vi "Inter Face.vi"() -> ()   [LabVIEW 2015]
uses:
  GUI_Control/Alarm.ctl
  GUI_Control/Home.ctl
  GUI_Control/Login.ctl
  GUI_Control/Manual.ctl
  GUI_Control/Open_data.ctl
  GUI_Control/Pause.ctl
  GUI_Control/Start.ctl
  GUI_Control/Stop.ctl
  GUI_Control/Inforamation_11.ctl
  <userlib>/QMH/Message Queue/Support/RunType.ctl
  <userlib>/QMH/Message Queue/Support/Enqueue Message (Single).vi
  <vilib>/Utility/error.llb/Error Cluster From Error Code.vi
  <userlib>/QMH/Message Queue/Support/Enqueue Message (Array).vi
  <userlib>/QMH/Message Queue/Support/Run Module(ref).vi
  <vilib>/ErrorRing/Error Ring.xnode
  <userlib>/QMH/User Event - Stop/User Event - Stop.lvlib
  <userlib>/QMH/Message Queue/Message Queue.lvlib
panel:
  out "输出数组":string[](array[string])
  out "权限":enum16{"学生", "老师"}(ring)
  out "Time":string
  out "Data":string
  in  "Machine Information":T1
  in  "Exit":T2
  in  "Start":T3 caption="进入Scada监控"
  in  "Pause":T4
  in  "OpenData":T5 caption="动作-告警监视"
  in  "Manual":T6 caption="遥信遥测监控"
  in  "User":T7 caption="用户操作"
  in  "HOME":T8 caption="进入待机界面"
  in  "Alarm Information":T9
  in  "HostThread":variant
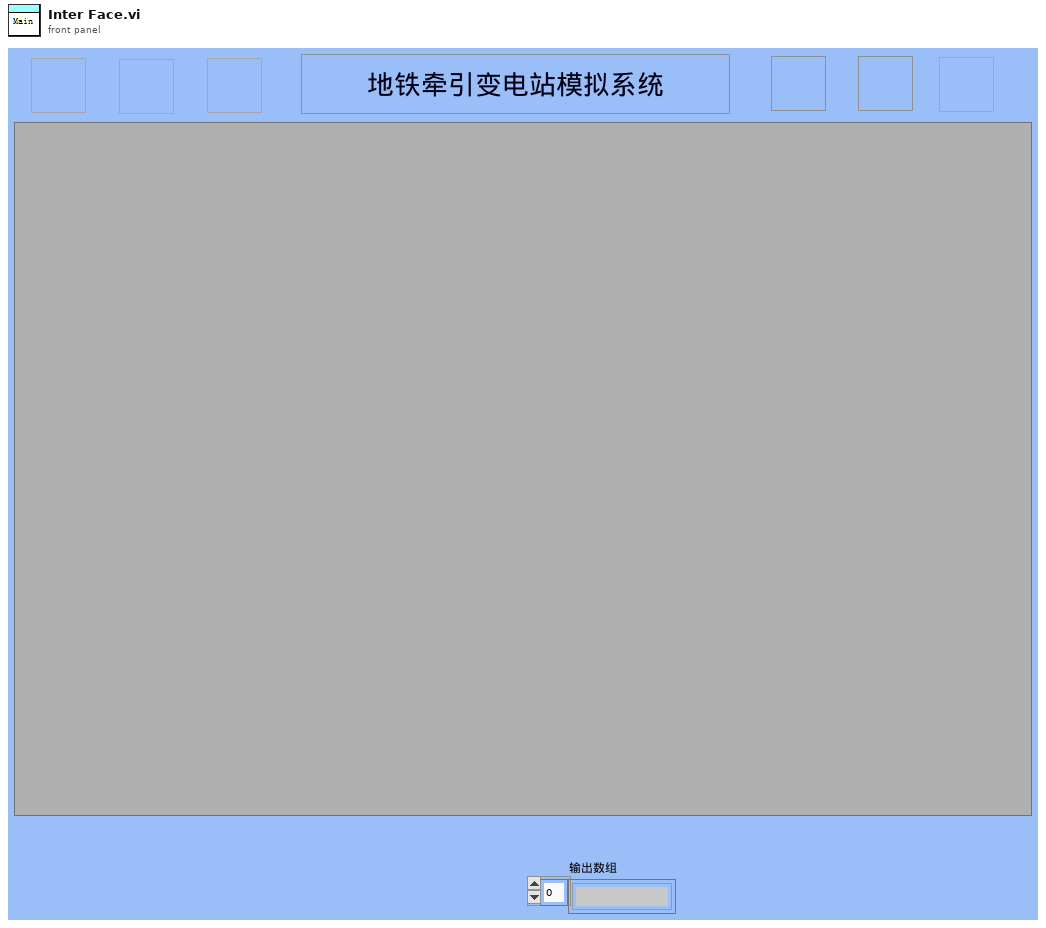
[diagram p1: front panel]
types:
  T1 = typedef "Inforamation_11.ctl" = bool
  T2 = typedef "Stop.ctl" = bool
  T3 = typedef "Start.ctl" = bool
  T4 = typedef "Pause.ctl" = bool
  T5 = typedef "Open_data.ctl" = bool
  T6 = typedef "Manual.ctl" = bool
  T7 = typedef "Login.ctl" = bool
  T8 = typedef "Home.ctl" = bool
  T9 = typedef "Alarm.ctl" = bool
  T10 = cluster{"Controls":cluster{"Exit":refnum<vi>, "Start":refnum<vi>, "Pause":refnum<vi>, "OpenData":refnum<vi>, "Machine Information":refnum<vi>, "Manual":refnum<vi>, "User":refnum<vi>, "HOME":refnum<vi>, "Alarm Information":refnum<vi>}, "Thread":cluster{"ThisQ":string, "ThisVI":refnum<vi>, "HostQ":string, "HostRef":refnum<vi>, "SlavesQ":string[], "SlavesRef":refnum<vi>[]}, "Data":cluster{"Replace":bool}, "User":cluster{"Name":string}, "子面板":refnum<vi>, " Authority":enum16{"学生", "老师"}}
  T11 = enum32{"Invalid", "Standard", "Closed", "Hidden", "Minimized", "Maximized"}
  T12 = typedef "Message Queue.lvlib/RunType.ctl" = enum16{"Embeded", "Standard", "Hidden", "Minimized", "Maximzed", "RealTime"}
  T13 = enum8{"Enabled", "Disabled", "Disabled and Grayed Out"}
  T14 = cluster{"Exit":refnum<vi>, "Start":refnum<vi>, "Pause":refnum<vi>, "OpenData":refnum<vi>, "Machine Information":refnum<vi>, "Manual":refnum<vi>, "User":refnum<vi>, "HOME":refnum<vi>, "Alarm Information":refnum<vi>}
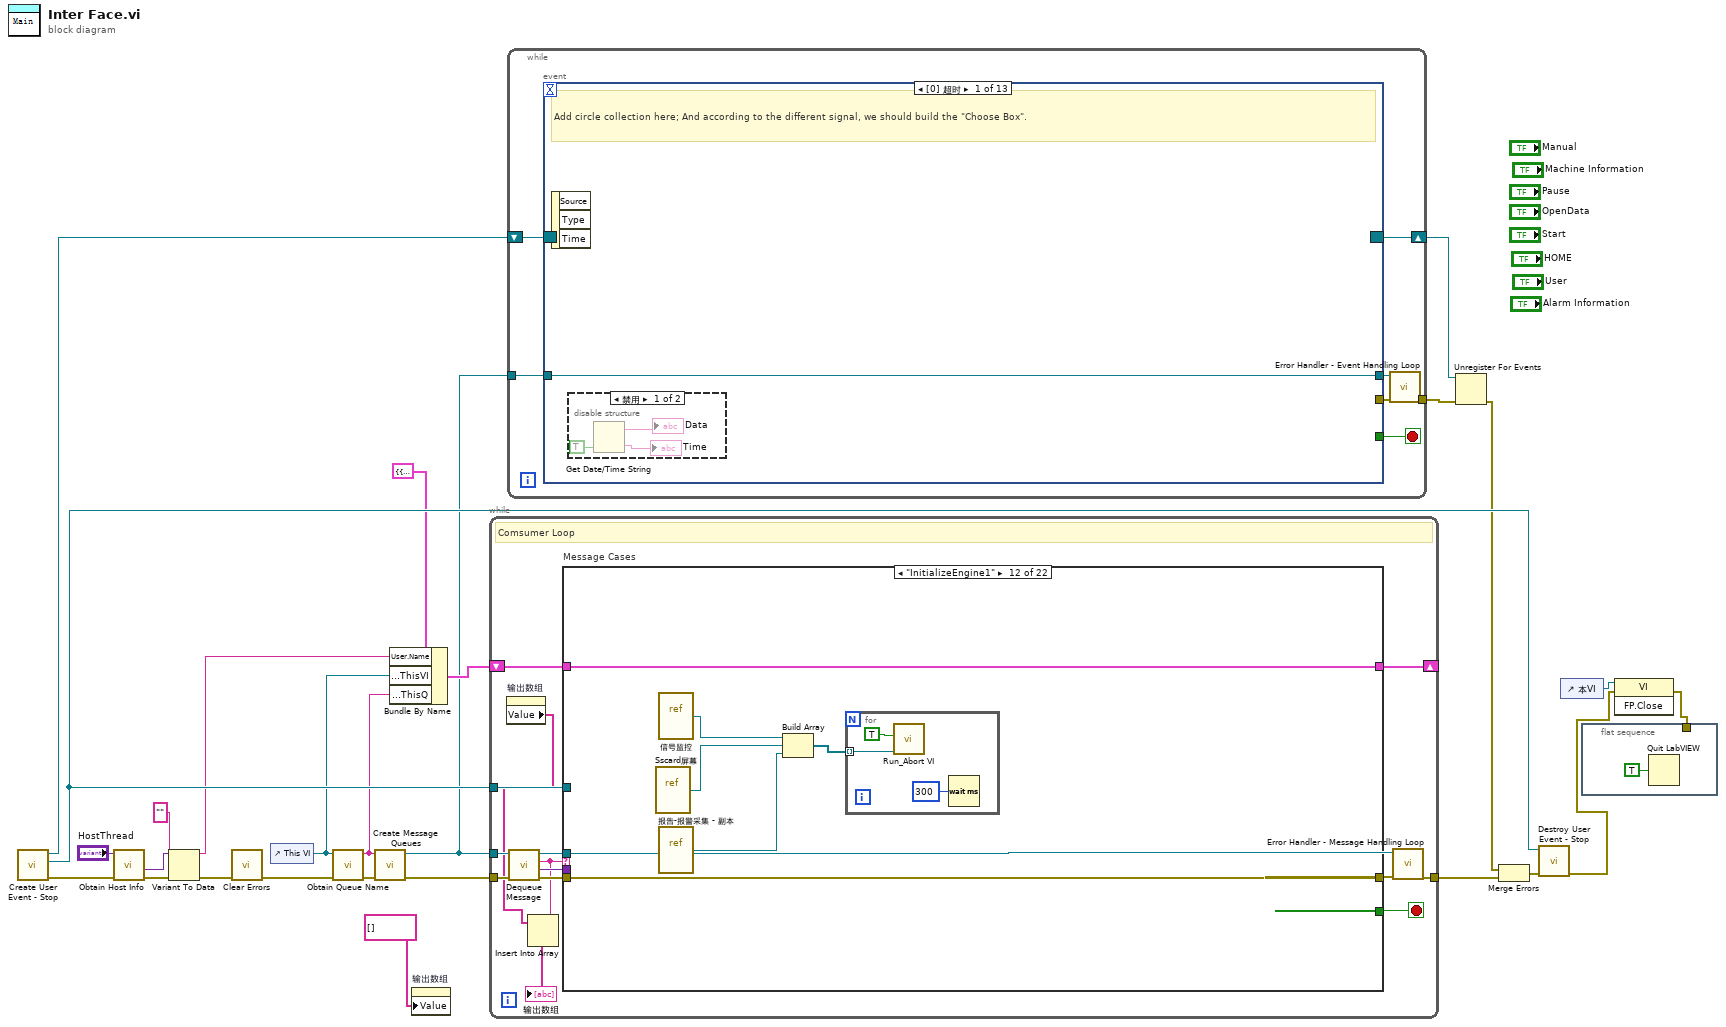
[diagram p0: block diagram]
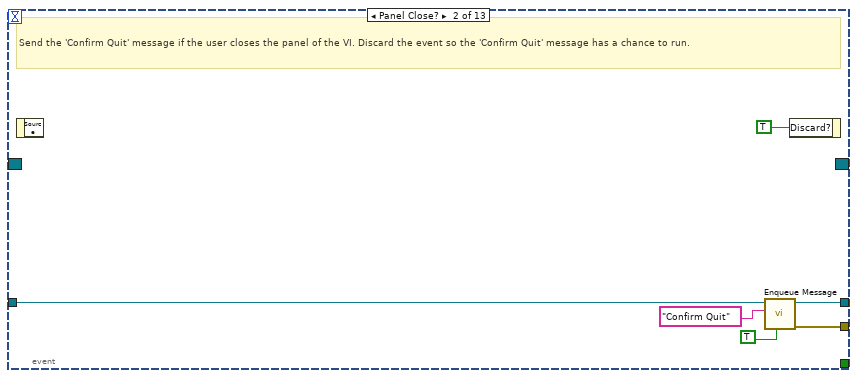
[diagram p3: hidden frame]
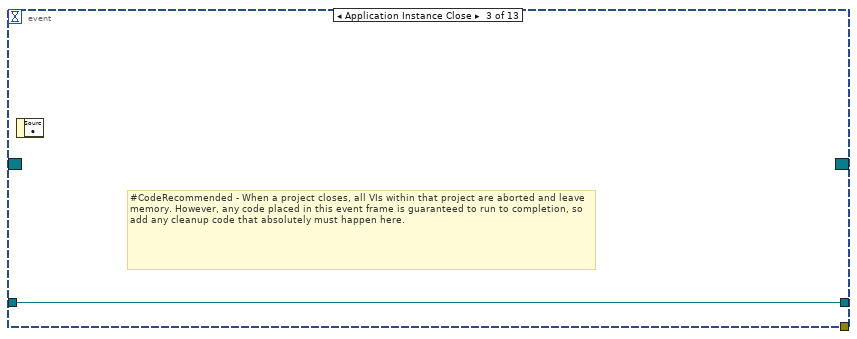
[diagram p4: hidden frame]
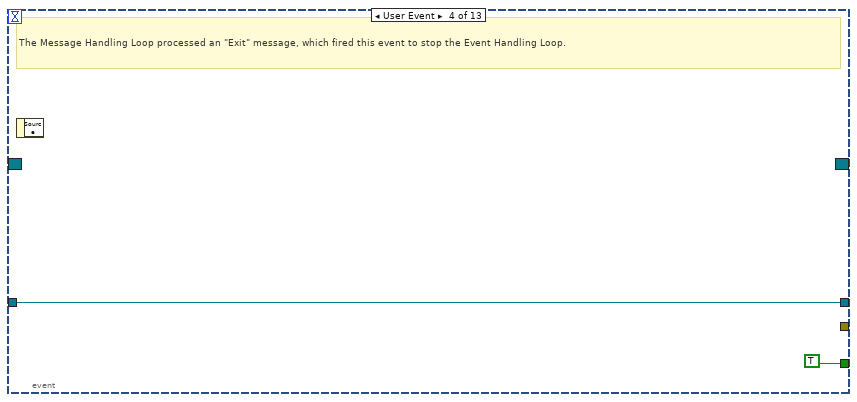
[diagram p5: hidden frame]
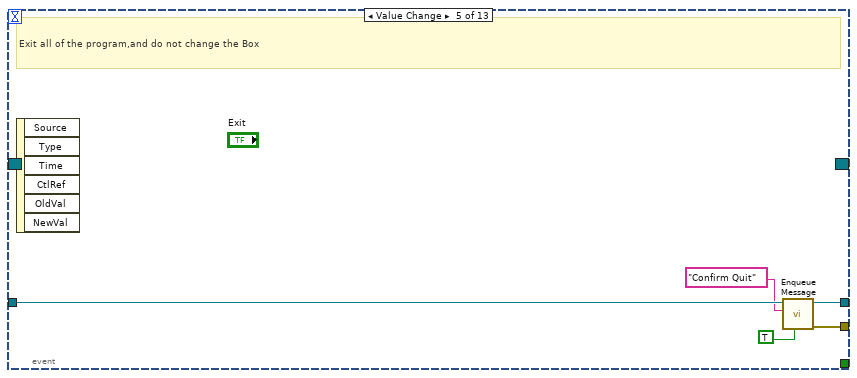
[diagram p6: hidden frame]
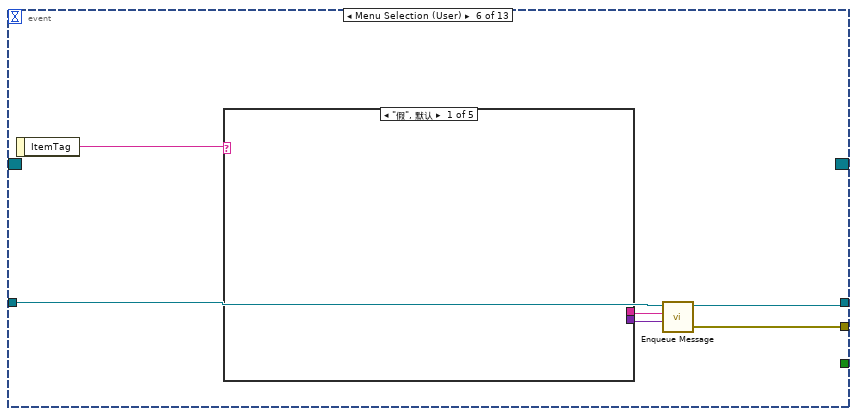
[diagram p7: hidden frame]
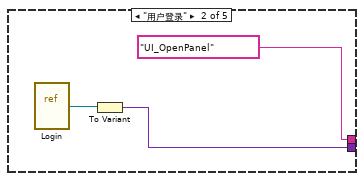
[diagram p8: hidden frame]
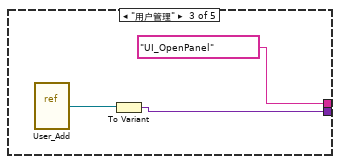
[diagram p9: hidden frame]
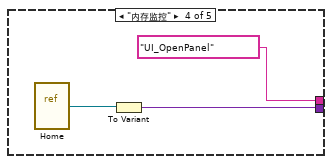
[diagram p10: hidden frame]
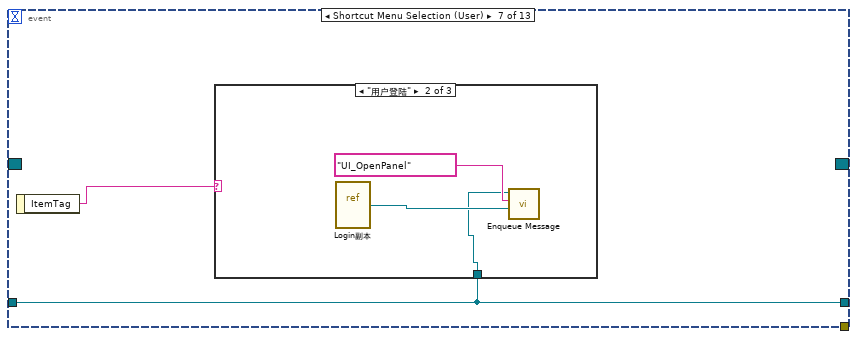
[diagram p12: hidden frame]
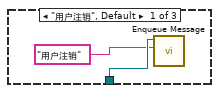
[diagram p13: hidden frame]
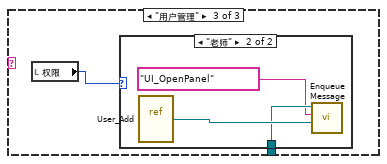
[diagram p14: hidden frame]
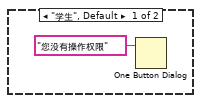
[diagram p15: hidden frame]
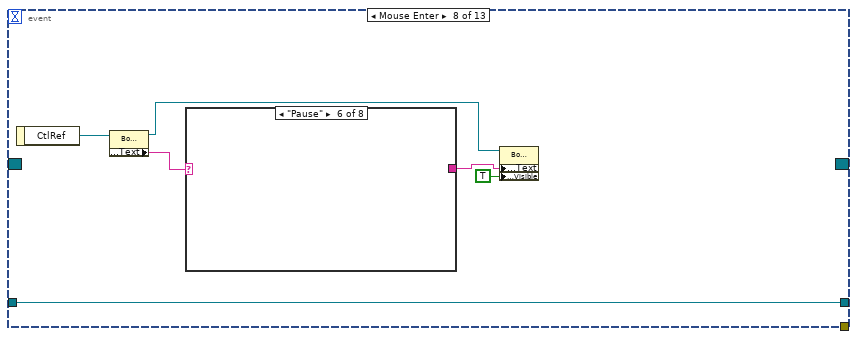
[diagram p16: hidden frame]
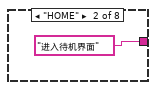
[diagram p18: hidden frame]
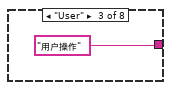
[diagram p19: hidden frame]
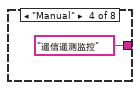
[diagram p20: hidden frame]
diagram:
  n1 = call <userlib>:"Create User Event - Stop.vi"() -> ("error out"=w14:errorcluster, "User Event - Stop"=w22:refnum<user-event>, "Stop Event Registration Refnum"=w24:refnum<event-registration>)  [unwired: 9 in]
  n2 = call <userlib>:"Obtain Host Info.vi"("error in (no error)"=w14, "HostThread"="HostThread") -> ("error out"=w11:errorcluster, "Data"=w10:variant)  [unwired: 6 in, 2 out]
  n3 = Variant To Data(error in=w11, type="", Variant=w10) -> (data=w6:string, error out=w8:errorcluster)
  n4 = call <vilib>:"Clear Errors.vi"("error in (no error)"=w8) -> ("error out"=w7:errorcluster)  [unwired: 5 in, 1 out]
  n5 = control-ref of="This VI"() -> (w5:refnum<vi>)
  n6 = call <userlib>:"Obtain Queue Name.vi"("error in (no error)"=w7, "VI Refnum"=w5) -> ("error out"=w18:errorcluster, "ViName"=w15:string)  [unwired: 8 in]
  n7 = call <userlib>:"Create Message Queues.vi"("error in (no error)"=w18, "name (unnamed)"=w15) -> ("error out"=w26:errorcluster, "QueueHandler"=w12:refnum<queue>)  [unwired: 8 in]
  n8 = Bundle By Name(cluster=T10 {"Controls"={"Exit"=refnum, "Start"=refnum, "Pause"=refnum, "OpenData"=refnum, "Machine Information"=refnum, "Manual"=refnum, "User"=refnum, "HOME"=refnum, "Alarm Information"=refnum}, "Thread"={"ThisQ"="", "ThisVI"=refnum, "HostQ"="", "HostRef"=refnum, "SlavesQ"=[], "SlavesRef"=[]}, "Data"={"Replace"=FALSE}, "User"={"Name"=""}, "子面板"=refnum, " Authority"=enum."学生"} ("Data Cluster"), "User.Name"=w6, "Thread.ThisVI"=w5, "Thread.ThisQ"=w15) -> (w16:T10)
  n9 = property on="输出数组" class="Arr (严格)"("Value"=string[] []) -> ()  [unwired: 2 in, 2 out]
  n10 = while {
    tunnel: w12 -> [w33]
    shift-right: [w39] -> _
    shift-left: w16 -> [w40]
    tunnel: w22 -> [w37]
    tunnel: w26 -> [w36]
    tunnel: [w31] -> w25
    stop <- w38 stop-if-true
    # "Comsumer Loop"
    n11 = property on="输出数组" class="Arr (严格)"() -> ("Value"=w27:string[])  [unwired: 2 in, 2 out]
    n12 = call <userlib>:"Dequeue Message.vi"("error in (no error)"=w36, "Message Queue"=w33) -> ("error out"=w35:errorcluster, "Message Data"=w34:variant, "Message"=w29:string, "dup Message Queue"=w32:refnum<queue>)  [unwired: 6 in]
    n13 = Insert Into Array(array=w27, new element=w29) -> (→"输出数组":string[])  [unwired: 1 in]
    n14 = case "Message Cases" shown="\"InitializeEngine1\"" w29 {
      selector: w29 -> [w41 _ _ _ _ _ _ _ _ _ _ _ _ _ _ _ _ _ _ _ _ _]
      tunnel: w32 -> [_ w59 _ w75 w89 _ w100 _ _ _ _ _ _ _ _ _ _ _ _ _ _ _]
      tunnel: w35 -> [_ w56 w73 w81 w87 w91 w102 w105 w111 w125 w137 w146 w151 w165 w177 w182 w193 w199 w201 w202 w205 w216]
      tunnel: [w42 w51 w68 w79 w88 w91 w101 w105 w111 w125 w137 w146 w151 w165 w177 w182 w193 w199 w201 w202 w205 w216] -> w30
      tunnel: w40 -> [w43 w53 w65 w80 w90 w92 w98 w104 w107 w124 w136 w145 w150 w164 w166 w181 w190 w196 w200 w203 w204 w215]
      tunnel: [w43 w53 w65 w80 w90 w92 w97 w104 w107 w124 w136 w145 w150 w163 w166 w181 w190 w196 w200 w203 w204 w215] -> w39
      tunnel: [_ TRUE _ _ _ _ _ _ _ _ _ _ _ _ _ _ _ _ _ _ _ _] -> w38
      tunnel: w34 -> [_ _ w72 _ _ _ w99 _ _ _ _ _ _ _ _ _ w192 w198 _ _ _ _]
      tunnel: w37 -> [_ w55 _ _ _ _ _ _ _ _ _ _ _ _ _ _ _ _ _ _ _ _]
      frame Default {
        # "'Default' case only runs if there is a message that isn't defined in any of the other cases.  Output a programming error."
        n15 = xnode "Error Ring"("参数 0"=w41) -> ("错误输出"=w42:errorcluster)
      }
      frame "Exit" {
        # "Stop the VI"
        # "Release the message queue reference"
        # "#CodeNeeded - Add any required cleanup code here"
        # "Exit - Exit the application."
        n16 = call <userlib>:"Fire User Event - Stop.vi"("User Event - Stop"=w55) -> ("error out"=w54:errorcluster)  [unwired: 10 in]
        n17 = Release Queue(queue=w59, error in (no error)=w56) -> (error out=w57:errorcluster)  [unwired: 1 in, 2 out]
        n18 = Merge Errors(w54, w57) -> (w51:errorcluster)
        n19 = call "Loop.vi"("Loop"=enum16{"Do Nothing", "Loop", "Stop"}."Stop") -> ()  [unwired: 4 in, 1 out]
      }
      frame "Error" {
        # "Error - Check the error message data and respond accordingly. This message is sent by the \"Error Handler\" VIs at the end of each loop in this application."
        n20 = Unbundle By Name(w65) -> ("Thread.HostQ"=w64:string)
        n21 = Variant To Data(error in=w73, type=errorcluster {"status"=FALSE, "code"=0, "source"=""} ("error constant"), Variant=w72) -> (data=w61:errorcluster, error out=w70:errorcluster)
        n22 = To Variant(anything=w61) -> (Variant=w60:variant)
        n23 = call <userlib>:"Obtain Message Queue.vi"("name (unnamed)"=w64) -> ("error out"=w63:errorcluster, "Message Queue"=w62:refnum<queue>)  [unwired: 9 in]
        n24 = call-poly <userlib>:"Enqueue Message.vi"("Priority Message? (F)"=TRUE, "error in (no error)"=w63, "Message Data"=w60, "Message"="Error", "Message Queue"=w62) -> ("error out"=w69:errorcluster)  [unwired: 5 in, 1 out]
        n25 = Merge Errors(w69, w70) -> (w68:errorcluster)
      }
      frame "Confirm Quit" {
        # "Confirm Quit - Message that can confirm whether or not the user wants to exit the application."
        n26 = for {
          tunnel: string[] ["Home.vi", "Sscard屏幕.vi", "AlarmInterFace.vi", "继保.vi", "测试接收队列.vi", "灯组解析.vi"] -> [w83] mode=indexing
          n27 = call <userlib>:"Obtain Message Queue.vi"("name (unnamed)"=w83) -> ("Message Queue"=w84:refnum<queue>)  [unwired: 9 in, 1 out]
          n28 = call-poly <userlib>:"Enqueue Message.vi"("Priority Message? (F)"=TRUE, "Message"="Exit", "Message Queue"=w84) -> ()  [unwired: 7 in, 2 out]
        }
        n29 = call-poly <userlib>:"Enqueue Message.vi"("Priority Message? (F)"=TRUE, "error in (no error)"=w81, "Message"="Exit", "Message Queue"=w75) -> ("error out"=w78:errorcluster)  [unwired: 6 in, 1 out]
        n30 = Merge Errors(w78) -> (w79:errorcluster)
      }
      frame "Initialize" {
        # "Initialize - Send separate messages to initialize the data and the front panel.  Bundle control references."
        n31 = call-poly <userlib>:"Enqueue Message.vi"("error in (no error)"=w87, "Message Array"=string[] ["UI_InitContorlRef", "UI_InitializePanel", "User_Initialize", "UI_InitContorlVal"], "Message Queue"=w89) -> ("error out"=w88:errorcluster)  [unwired: 7 in, 1 out]
      }
      frame "<-------User-------->" {
      }
      frame "User_Initialize" {
        w94 = enum16{"学生", "老师"}."学生"  # Authority
        n32 = Variant To Data(type=w94, Variant=w99) -> (data=w93:enum16{"学生", "老师"}, error out=w96:errorcluster)  [unwired: 1 in]
        "权限" <- w93
        n33 = call <vilib>:"Clear Errors.vi"("error in (no error)"=w96) -> ()  [unwired: 5 in, 2 out]
        n34 = Bundle By Name(cluster=w98, "Authority"=w93) -> (w97:T10)
        n35 = call "Loop.vi"("Loop"=enum16{"Do Nothing", "Loop", "Stop"}."Loop") -> ()  [unwired: 4 in, 1 out]
        n36 = call-poly <userlib>:"Enqueue Message.vi"("error in (no error)"=w102, "Message Array"=string[] ["User_Wirte authority", "User_update authority1", "User_update authority2", "InitializeEngine", "InitializeEngine1"], "Message Queue"=w100) -> ("error out"=w101:errorcluster)  [unwired: 7 in, 1 out]
      }
      frame "User_Wirte authority" {
      }
      frame "User_update authority1" {
        n37 = Unbundle By Name(w107) -> ("Authority"=w106:enum16{"学生", "老师"})
        n38 = case shown="\"学生\", 默认" w106 {
          tunnel: [bool[] [FALSE] _] -> w109
          frame "学生", Default {
          }
          frame "老师" {
          }
        }
        n39 = Current VI's Menubar() -> (w110:refnum<k9>)
        n40 = for {
          tunnel: w110 -> [w114]
          tunnel: w109 -> [w113] mode=indexing
          tunnel: string[] ["用户管理"] -> [w112] mode=indexing
          n41 = Set Menu Item Info(7:w112, 9:w113, 10:w112, 11:w114) -> ()  [unwired: 3 in, 2 out]
        }
      }
      frame "User_update authority2" {
        n42 = Unbundle By Name(w124) -> ("Controls.Exit"=w118:refnum<vi>, "Controls.OpenData"=w123:refnum<vi>, "Controls.HOME"=w122:refnum<vi>, "Controls.Manual"=w121:refnum<vi>, "Controls.Start"=w117:refnum<vi>, "Authority"=w116:enum16{"学生", "老师"})
        n43 = Build Array(w118, w123, w122, w121, w117) -> (w120:refnum<vi>[])
        n44 = case shown="\"学生\", 默认" w116 {
          tunnel: [i32[] [2, 2, 2, 2, 0] i32[] [0, 0, 0, 0, 0]] -> w119
          frame "学生", Default {
          }
          frame "老师" {
          }
        }
        n45 = for {
          tunnel: w120 -> [w127] mode=indexing
          tunnel: w119 -> [w126] mode=indexing
          n46 = property class="Bool"(reference=w127, "DisabledEnum"=w126) -> ()  [unwired: 1 in, 2 out]
        }
      }
      frame "InitializeEngine" {
        n47 = vi-ref "管理机.vi"() -> (w135:refnum<vi>)
        n48 = vi-ref "继保.vi"() -> (w133:refnum<vi>)
        n49 = vi-ref "OPC.vi"() -> (w132:refnum<vi>)
        n50 = vi-ref "测试接收队列.vi"() -> (w131:refnum<vi>)
        n51 = vi-ref "灯组解析.vi"() -> (w130:refnum<vi>)
        n52 = Build Array(w135, w133, w132, w131, w130) -> (w134:refnum<vi>[])
        n53 = for {
          tunnel: w134 -> [w139] mode=indexing
          n54 = call "Run_Abort VI.vi"("VI引用句柄"=w139, "Run?(Default Abort)"=TRUE) -> ()  [unwired: 10 in]
          n55 = Wait (ms)(milliseconds to wait=u32 300 ("等待时间（毫秒）")) -> ()  [unwired: 1 out]
        }
      }
      frame "InitializeEngine1" {
        n56 = vi-ref "Sscard屏幕.vi"() -> (w142:refnum<vi>)
        n57 = vi-ref "信号监控.vi"() -> (w143:refnum<vi>)
        n58 = vi-ref "报告-报警采集 - 副本.vi"() -> (w141:refnum<vi>)
        n59 = Build Array(w143, w142, w141) -> (w144:refnum<vi>[])
        n60 = for {
          tunnel: w144 -> [w148] mode=indexing
          n61 = call "Run_Abort VI.vi"("VI引用句柄"=w148, "Run?(Default Abort)"=TRUE) -> ()  [unwired: 10 in]
          n62 = Wait (ms)(milliseconds to wait=u32 300 ("等待时间（毫秒）")) -> ()  [unwired: 1 out]
        }
      }
      frame "<-------UI-------->" {
      }
      frame "UI_InitContorlRef" {
        n63 = control-ref of="Exit"() -> (w162:refnum<vi>)
        n64 = control-ref of="Start"() -> (w161:refnum<vi>)
        n65 = control-ref of="Pause"() -> (w160:refnum<vi>)
        n66 = control-ref of="HOME"() -> (w155:refnum<vi>)
        n67 = control-ref of="Alarm Information"() -> (w154:refnum<vi>)
        n68 = control-ref of="OpenData"() -> (w159:refnum<vi>)
        n69 = control-ref of="Manual"() -> (w157:refnum<vi>)
        n70 = control-ref of="User"() -> (w156:refnum<vi>)
        n71 = control-ref of="Machine Information"() -> (w158:refnum<vi>)
        n72 = Bundle("Exit"=w162, "Start"=w161, "Pause"=w160, "OpenData"=w159, "Machine Information"=w158, "Manual"=w157, "User"=w156, "HOME"=w155, "Alarm Information"=w154) -> (w153:T14)  [unwired: 1 in]
        n73 = control-ref of="子面板"() -> (w152:refnum<vi>)
        n74 = Bundle By Name(cluster=w164, "Controls"=w153, "子面板"=w152) -> (w163:T10)
      }
      frame "UI_InitContorlVal" {
        # "初始化控件值"
        n75 = Unbundle By Name(w166) -> ("Controls.Machine Information"=w175:refnum<vi>, "Controls.Exit"=w174:refnum<vi>, "Controls.Start"=w173:refnum<vi>, "Controls.Pause"=w172:refnum<vi>, "Controls.OpenData"=w171:refnum<vi>, "Controls.Manual"=w170:refnum<vi>, "Controls.User"=w169:refnum<vi>, "Controls.HOME"=w168:refnum<vi>)
        n76 = Build Array(w174, w173, w172, w171, w170, w169, w168) -> (w167:refnum<vi>[])
        n77 = for {
          tunnel: w167 -> [w178] mode=indexing
          n78 = invoke class="Bool" method="Reinit To Default"(reference=w178) -> ()  [unwired: 2 in, 3 out]
        }
        n79 = property class="Bool (严格)"(reference=w175, "BoolText.Text"="地铁牵引变电站模拟系统" ("布尔文本.文本")) -> ()  [unwired: 1 in, 2 out]
      }
      frame "UI_InitializePanel" {
        # "加载初始子面板VI"
        n80 = Unbundle By Name(w181) -> ("子面板"=w180:refnum<vi>)
        n81 = vi-ref "Home.vi"() -> (w179:refnum<vi>)
        n82 = call "Serch.vi"("静态VI"=w179, "子面板"=w180) -> ()  [unwired: 2 in]
      }
      frame "UI_OpenPanel" {
        # "运行VI，如果状态为运行，打开前面板， 在子VI中设置退出时候是否结束程序"
        n83 = Variant To Data(type=refnum<vi> refnum, Variant=w192) -> (data=w189:refnum<vi>)  [unwired: 1 in, 1 out]
        n84 = call-poly <userlib>:"Run Module.vi"("Type"=RunType."Standard", "VI Ref in"=w189) -> ("VI Ref out"=w183:refnum<vi>)  [unwired: 7 in, 2 out]
        n85 = invoke class="VI" method="FP.Open"(reference=w183, "Activate"=TRUE ("激活？"), "State"=T11."Standard" ("状态")) -> (reference out=w187:refnum<vi>)  [unwired: 2 in, 4 out]
        n86 = property class="VI"(reference=w187, "Front Panel.IsFrontmost"=TRUE ("前面板窗口:在最前")) -> ()  [unwired: 1 in, 2 out]
      }
      frame "UI_insertPanel" {
        # "VI插入子面板"
        n87 = Unbundle By Name(w196) -> ("子面板"=w195:refnum<vi>)
        n88 = Variant To Data(type=refnum<vi> refnum, Variant=w198) -> (data=w194:refnum<vi>)  [unwired: 1 in, 1 out]
        n89 = call "Serch.vi"("静态VI"=w194, "子面板"=w195) -> ()  [unwired: 2 in]
      }
      frame "<------Core------>" {
      }
      frame "Core_InitializeRef" {
        # "Initialize control references. For there is not enough space to locate all the control references, separate the codes into 2 messages"
      }
      frame "<---Operation--->" {
      }
      frame "用户注销" {
        n90 = Unbundle By Name(w215) -> ("Controls.OpenData"=w212:refnum<vi>, "Controls.Manual"=w211:refnum<vi>, "Controls.Alarm Information"=w210:refnum<vi>, "Controls.Start"=w209:refnum<vi>, "子面板"=w207:refnum<vi>)
        n91 = vi-ref "Home.vi"() -> (w208:refnum<vi>)
        n92 = Build Array(w212, w211, w210, w209) -> (w214:refnum<vi>[])
        n93 = call "Serch.vi"("静态VI"=w208, "子面板"=w207) -> ()  [unwired: 2 in]
        n94 = for {
          tunnel: w214 -> [w218] mode=indexing
          tunnel: T13."Disabled and Grayed Out" ("禁用") -> [w217]
          n95 = property class="Bool (严格)"(reference=w218, "DisabledEnum"=w217) -> ()  [unwired: 1 in, 2 out]
        }
        n96 = local write "权限"(enum16{"学生", "老师"}."学生" ("权限")) -> ()
      }
    }
    n97 = call <userlib>:"Error Handler - Message Handling Loop.vi"("error in (no error)"=w30, "Message Queue"=w32) -> ("dup error in"=w31:errorcluster)  [unwired: 8 in, 1 out]
  }
  n98 = while {
    tunnel: w12 -> [w225]
    shift-right: [w223] -> w20
    shift-left: w24 -> [w224]
    tunnel: [w219] -> w19
    stop <- w221 stop-if-true
    # "Producer Loop"
    n99 = event shown="[0] 超时" {
      selector: w224 -> [_ _ _ _ _ _ _ _ _ _ _ _ _]
      dyn-events: [_ _ _ _ _ _ _ _ _ _ _ _ _] -> w223
      timeout: _ -> [_ _ _ _ _ _ _ _ _ _ _ _ _]
      tunnel: [_ _ _ TRUE ("Discard?") _ _ _ _ _ _ _ _ _] -> w221
      tunnel: w225 -> [w226 w234 w236 w238 w243 w247 w259 w277 w285 w289 w298 w307 w316]
      tunnel: [_ w233 _ _ w241 w248 _ _ _ _ _ _ _] -> w222
      tunnel: [w226 w232 w236 w238 w242 w249 w259 w277 w285 w288 w297 w305 w315] -> w220
      event Timeout {
        # "Add circle collection here; And according to the different signal, we should build the \"Choose Box\"."
        n100 = event-data() -> ()  [unwired: 1 in, 3 out]
        n101 = disable-structure shown="禁用" {
          frame Disabled {
            n102 = Get Date/Time String(want seconds? (F)=TRUE ("需要秒？(F)")) -> (date string=→"Data":string, time string=→"Time":string)  [unwired: 2 in]
          }
          frame Enabled {
          }
        }
      }
      event Panel Close? {
        # "Send the 'Confirm Quit' message if the user closes the panel of the VI. Discard the event so the 'Confirm Quit' message has a chance to run."
        n103 = event-data() -> ()  [unwired: 1 in, 1 out]
        n104 = call-poly <userlib>:"Enqueue Message.vi"("Priority Message? (F)"=TRUE, "Message"="Confirm Quit", "Message Queue"=w234) -> ("error out"=w233:errorcluster, "dup Message Queue"=w232:refnum<queue>)  [unwired: 7 in]
        n105 = event-data("Discard?"=TRUE) -> ()  [unwired: 1 in, 1 out]
      }
      event Application Instance Close {
        # "#CodeRecommended - When a project closes, all VIs within that project are aborted and leave memory. However, any code placed in this event frame is guaranteed to run to completion, so add any cleanup code that absolutely must happen here."
        n106 = event-data() -> ()  [unwired: 1 in, 1 out]
      }
      event User Event {
        # "The Message Handling Loop processed an \"Exit\" message, which fired this event to stop the Event Handling Loop."
        n107 = event-data() -> ()  [unwired: 1 in, 1 out]
      }
      event Value Change {
        # "Exit all of the program,and do not change the Box"
        n108 = event-data() -> ()  [unwired: 1 in, 6 out]
        n109 = call-poly <userlib>:"Enqueue Message.vi"("Priority Message? (F)"=TRUE, "Message"="Confirm Quit", "Message Queue"=w243) -> ("error out"=w241:errorcluster, "dup Message Queue"=w242:refnum<queue>)  [unwired: 7 in]
      }
      event Menu Selection (User) {
        n110 = event-data() -> ("ItemTag"=w245:string)  [unwired: 1 in]
        n111 = case shown="\"假\", 默认" w245 {
          tunnel: [_ "UI_OpenPanel" "UI_OpenPanel" "UI_OpenPanel" _] -> w246
          tunnel: [_ w250 w253 w256 _] -> w244
          frame "假", Default {
          }
          frame "用户登录" {
            n112 = vi-ref "Login.vi"() -> (w252:refnum<vi>)
            n113 = To Variant(anything=w252) -> (Variant=w250:variant)
          }
          frame "用户管理" {
            n114 = vi-ref "User_Add.vi"() -> (w255:refnum<vi>)
            n115 = To Variant(anything=w255) -> (Variant=w253:variant)
          }
          frame "内存监控" {
            n116 = vi-ref "Home.vi"() -> (w257:refnum<vi>)
            n117 = To Variant(anything=w257) -> (Variant=w256:variant)
          }
          frame "注销登陆" {
          }
        }
        n118 = call-poly <userlib>:"Enqueue Message.vi"("Message Data"=w244, "Message"=w246, "Message Queue"=w247) -> ("error out"=w248:errorcluster, "dup Message Queue"=w249:refnum<queue>)  [unwired: 7 in]
      }
      event Shortcut Menu Selection (User) {
        n119 = event-data() -> ("ItemTag"=w260:string)  [unwired: 1 in]
        n120 = case shown="\"用户登陆\"" w260 {
          tunnel: w259 -> [w262 w263 w267]
          frame "用户注销", Default {
            n121 = call-poly <userlib>:"Enqueue Message.vi"("Message"="用户注销", "Message Queue"=w262) -> ()  [unwired: 8 in, 2 out]
          }
          frame "用户登陆" {
            n122 = vi-ref "Login副本.vi"() -> (w265:refnum<vi>)
            n123 = call-poly <userlib>:"Enqueue Message.vi"("Message Data"=w265, "Message"="UI_OpenPanel", "Message Queue"=w263) -> ()  [unwired: 7 in, 2 out]
          }
          frame "用户管理" {
            n124 = local read "权限"() -> (w266:enum16{"学生", "老师"})
            n125 = case shown="\"老师\"" w266 {
              tunnel: w267 -> [_ w270]
              frame "学生", Default {
                n126 = One Button Dialog(message="您没有操作权限" ("消息")) -> ()  [unwired: 1 in, 1 out]
              }
              frame "老师" {
                n127 = vi-ref "User_Add.vi"() -> (w271:refnum<vi>)
                n128 = call-poly <userlib>:"Enqueue Message.vi"("Message Data"=w271, "Message"="UI_OpenPanel", "Message Queue"=w270) -> ()  [unwired: 7 in, 2 out]
              }
            }
          }
        }
      }
      event Mouse Enter {
        n129 = event-data() -> ("CtlRef"=w276:refnum<vi>)  [unwired: 1 in]
        n130 = property class="Bool (严格)"(reference=w276) -> (reference out=w274:refnum<vi>, "Label.Text"=w275:string)  [unwired: 1 in, 1 out]
        n131 = case shown="\"Pause\"" w275 {
          tunnel: [_ "进入待机界面" "用户操作" "遥信遥测监控" "进入Scada监控" _ _ "动作-告警监视"] -> w273
          frame "假", Default {
          }
          frame "HOME" {
          }
          frame "User" {
          }
          frame "Manual" {
          }
          frame "Start" {
          }
          frame "Pause" {
          }
          frame "Exit" {
          }
          frame "OpenData" {
          }
        }
        n132 = property class="Bool (严格)"(reference=w274, "Caption.Text"=w273, "Caption.Visible"=TRUE ("标题.可见")) -> ()  [unwired: 1 in, 2 out]
      }
      event Mouse Leave {
        n133 = event-data() -> ("CtlRef"=w283:refnum<vi>)  [unwired: 1 in]
        n134 = property class="Bool (严格)"(reference=w283, "Caption.Visible"=FALSE ("标题.可见")) -> ()  [unwired: 1 in, 2 out]
      }
      event Value Change {
        n135 = event-data() -> ("CtlRef"=w286:refnum<vi>, "NewVal"=w287:T6)  [unwired: 1 in]
        n136 = invoke on="调用节点" class="Bool (严格)" method="Reinit To Default"(reference=w286) -> ()  [unwired: 2 in, 3 out]
        n137 = case shown="真" w287 {
          tunnel: w289 -> [w290 w294]
          tunnel: [w290 w293] -> w288
          frame False {
          }
          frame True {
            n138 = vi-ref "信号监控.vi"() -> (w291:refnum<vi>)
            n139 = call-poly <userlib>:"Enqueue Message.vi"("Message Data"=w291, "Message"="UI_insertPanel", "Message Queue"=w294) -> ("dup Message Queue"=w293:refnum<queue>)  [unwired: 7 in, 1 out]
          }
        }
      }
      event Value Change {
        n140 = event-data() -> ("CtlRef"=w296:refnum<vi>, "NewVal"=w295:T5)  [unwired: 1 in]
        n141 = invoke on="调用节点" class="Bool (严格)" method="Reinit To Default"(reference=w296) -> ()  [unwired: 2 in, 3 out]
        n142 = case shown="假" w295 {
          tunnel: w298 -> [w299 w303]
          tunnel: [w299 w302] -> w297
          frame False {
          }
          frame True {
            n143 = vi-ref "测试接收队列.vi"() -> (w300:refnum<vi>)
            n144 = call-poly <userlib>:"Enqueue Message.vi"("Message Data"=w300, "Message"="UI_insertPanel", "Message Queue"=w303) -> ("dup Message Queue"=w302:refnum<queue>)  [unwired: 7 in, 1 out]
          }
        }
      }
      event Value Change {
        n145 = event-data() -> ("CtlRef"=w304:refnum<vi>, "NewVal"=w306:T3)  [unwired: 1 in]
        n146 = invoke on="调用节点" class="Bool (严格)" method="Reinit To Default"(reference=w304) -> ()  [unwired: 2 in, 3 out]
        n147 = case shown="假" w306 {
          tunnel: w307 -> [w312 w313]
          tunnel: [w308 w313] -> w305
          frame True {
            n148 = vi-ref "Sscard屏幕.vi"() -> (w309:refnum<vi>)
            n149 = To Variant(anything=w309) -> (Variant=w311:variant)
            n150 = call-poly <userlib>:"Enqueue Message.vi"("Message Data"=w311, "Message"="UI_insertPanel", "Message Queue"=w312) -> ("dup Message Queue"=w308:refnum<queue>)  [unwired: 7 in, 1 out]
          }
          frame False {
          }
        }
      }
      event Value Change {
        n151 = event-data() -> ("CtlRef"=w314:refnum<vi>, "NewVal"=w317:T8)  [unwired: 1 in]
        n152 = invoke class="Bool (严格)" method="Reinit To Default"(reference=w314) -> ()  [unwired: 2 in, 3 out]
        n153 = case shown="真" w317 {
          tunnel: w316 -> [w318 w321]
          tunnel: [w318 w320] -> w315
          frame False {
          }
          frame True {
            n154 = call-poly <userlib>:"Enqueue Message.vi"("Message"="UI_InitializePanel", "Message Queue"=w321) -> ("dup Message Queue"=w320:refnum<queue>)  [unwired: 8 in, 1 out]
          }
        }
      }
    }
    n155 = call <userlib>:"Error Handler - Event Handling Loop.vi"("error in (no error)"=w222, "Message Queue"=w220) -> ("dup error in"=w219:errorcluster)  [unwired: 8 in, 1 out]
  }
  n156 = Unregister For Events(event registration refnum=w20, error in=w19) -> (error out=w21:errorcluster)
  n157 = Merge Errors(w21, w25) -> (w23:errorcluster)
  n158 = call <userlib>:"Destroy User Event - Stop.vi"("error in (no error)"=w23, "User Event - Stop"=w22) -> ("error out"=w3:errorcluster)  [unwired: 9 in]
  n159 = control-ref of="本VI"() -> (w4:refnum<vi>)
  n160 = flat-sequence {
    tunnel: w2 -> [_]
    frame #0 {
      n161 = Quit LabVIEW(quit? (T)=TRUE ("退出？(T)")) -> ()
    }
  }
  n162 = invoke class="VI" method="FP.Close"(reference=w4, error in=w3) -> (error out=w2:errorcluster)  [unwired: 1 in, 2 out]
